vi "Insert Subsequence.vi"(8 "error in (no error)":errorcluster, 10 "Insert Subsequence":T1, 11 "Test Executive Builder in":refnum<class "Test Executive Builder.lvclass">) -> (0 "error out":errorcluster, 3 "Test Executive Builder out":refnum<class "Test Executive Builder.lvclass">, 5 "Unique ID out":string)   [LabVIEW 2017, in "Test Executive Builder.lvclass"]
uses:
  Test Executive Builder.lvclass
  Source/Test Executive Builder Model/Test Executive Builder Model/Test Executive Builder Model.lvclass
  c6fbb65b-fd05-43f5-9c36-3c85fd8e5414.vi
  C:/Users/jonmc/Documents/Git/Test Executive Builder/Source/Test Executive Builder Model/Test Executive Builder Model/Test Executive Builder Model.lvclass
  C:/Users/jonmc/Documents/Git/Test Executive Builder/gpm_packages/@cs/mva-core/Source/IModel/IModel/IModel.lvclass
  <vilib>/gpm_packages/@cs/mva-core/Source/IModel/IModel/IModel.lvclass
  Source/Test Executive Builder Dialogs/ITest Executive Builder Dialog/ITest Executive Builder Dialog.lvclass
  Source/Application Dependencies/Insert Subsequence.ctl
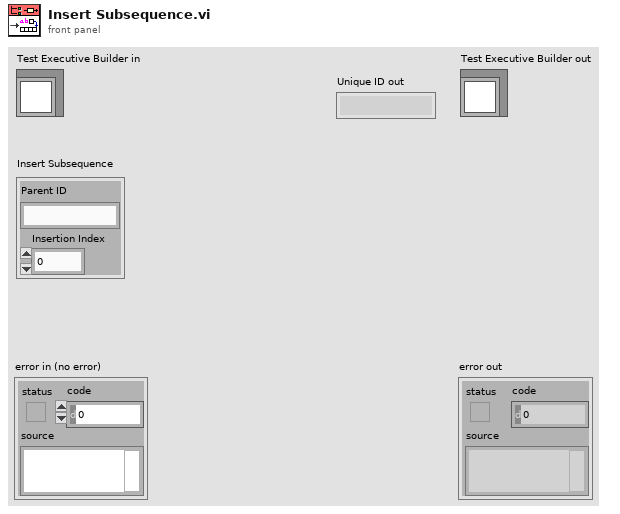
[diagram p1: front panel]
types:
  T1 = typedef "Insert Subsequence.ctl" = cluster{"Parent ID":string, "Insertion Index":i32}
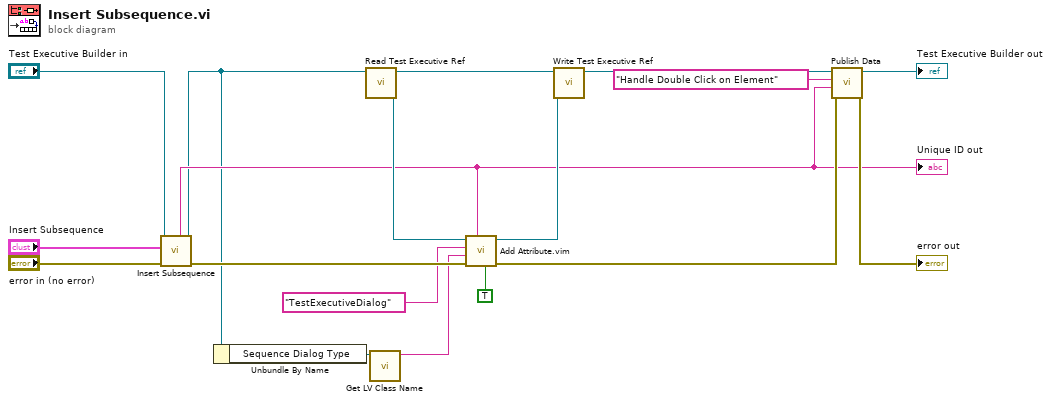
[diagram p0: block diagram]
diagram:
  n1 = call-parent "Insert Subsequence.vi"("error in (no error)"="error in (no error)", "Insert Subsequence"="Insert Subsequence", "Test Executive Builder Model in"="Test Executive Builder in") -> ("error out"=w14:errorcluster, "Test Executive Builder Model out"=w2:refnum<class "Test Executive Builder.lvclass">, "Unique ID out"=w3:string)  [unwired: 6 in]
  "Unique ID out" <- w3
  n2 = Unbundle By Name(w2) -> ("Sequence Dialog Type"=w1:refnum<class "ITest Executive Builder Dialog.lvclass">)
  n3 = call "Read Test Executive Ref.vi"("Test Executive Builder Model in"=w2) -> ("Test Executive Ref"=w13:refnum<data-value>, "Test Executive Builder Model out"=w15:refnum<class "Test Executive Builder.lvclass">)  [unwired: 9 in]
  n4 = call <vilib>:"Get LV Class Name.vi"("object"=w1) -> ("class name"=w9:string)  [unwired: 9 in, 1 out]
  n5 = call "Add Attribute.vim"("Private?"=TRUE, "ID"=w3, "error in (no error)"=w14, "Attribute"=w9, "Attribute Name"="TestExecutiveDialog", "Test Executive Ref"=w13) -> ("error out"=w5:errorcluster, "Test Executive Ref out"=w12:refnum<data-value>)  [unwired: 2 in, 2 out]
  n6 = call "Write Test Executive Ref.vi"("Test Executive Ref"=w12, "Test Executive Builder Model in"=w15) -> ("Test Executive Builder Model out"=w7:refnum<class "Test Executive Builder.lvclass">)  [unwired: 9 in]
  n7 = call <vilib>:"Publish Data.vi"("error in (no error)"=w5, "Data to Publish"=w3, "Datum Name"="Handle Double Click on Element", "IModel in"=w7) -> ("error out"=→"error out":errorcluster, "IModel out"=→"Test Executive Builder out":refnum<class "Test Executive Builder.lvclass">)  [unwired: 6 in]
